vi "Add LVClass to Lib.vi"(8 "error in (no error)":errorcluster, 10 "LVClass Path in":path, 11 "Library in":refnum<vi>) -> (0 "error out":errorcluster, 2 "LVClassLibrary out":refnum<vi>, 3 "Library out":refnum<vi>)   [LabVIEW 2019, in "gRPC Template Creation Utility.lvlib"]
uses:
  gRPC Template Creation Utility.lvlib
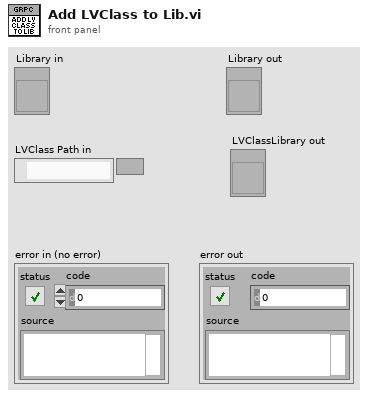
[diagram p1: front panel]
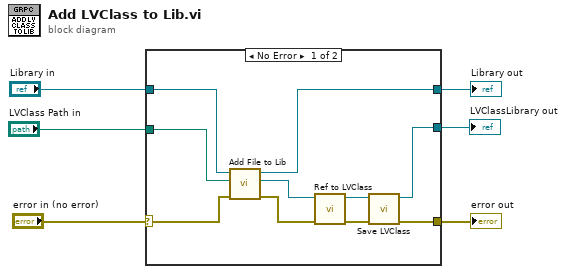
[diagram p0: block diagram]
diagram:
  n1 = case shown="No Error" "error in (no error)" {
    selector: "error in (no error)" -> [w7 w17]
    tunnel: [w16 w17] -> w6
    tunnel: "LVClass Path in" -> [w11 _]
    tunnel: [w10 w18] -> w4
    tunnel: "Library in" -> [w9 w18]
    tunnel: [w8 _] -> w2
    frame No Error {
      n2 = call "Add File to Lib.vi"("error in (no error)"=w7, "File Path"=w11, "Library in"=w9) -> ("error out"=w14:errorcluster, "File Ref"=w12:refnum<vi>, "Library out"=w10:refnum<vi>)  [unwired: 6 in]
      n3 = call "Ref to LVClass.vi"("error in (no error)"=w14, "ProjectItem in"=w12) -> ("error out"=w15:errorcluster, "LVClassLibrary out"=w13:refnum<vi>)  [unwired: 8 in]
      n4 = call "Save LVClass.vi"("error in (no error)"=w15, "LVClassLibrary in"=w13) -> ("error out"=w16:errorcluster, "LVClassLibrary out"=w8:refnum<vi>)  [unwired: 8 in]
    }
    frame Error {
    }
  }
  "error out" <- w6
  "Library out" <- w4
  "LVClassLibrary out" <- w2
